vi "save.vi"(0 "ItemNames":string[][](array[string])) -> ()   [LabVIEW 2020]
uses:
  <vilib>/Utility/file.llb/Write Delimited Spreadsheet (string).vi
panel:
  out "Array":string[][](array[string])
  out "error out":errorcluster
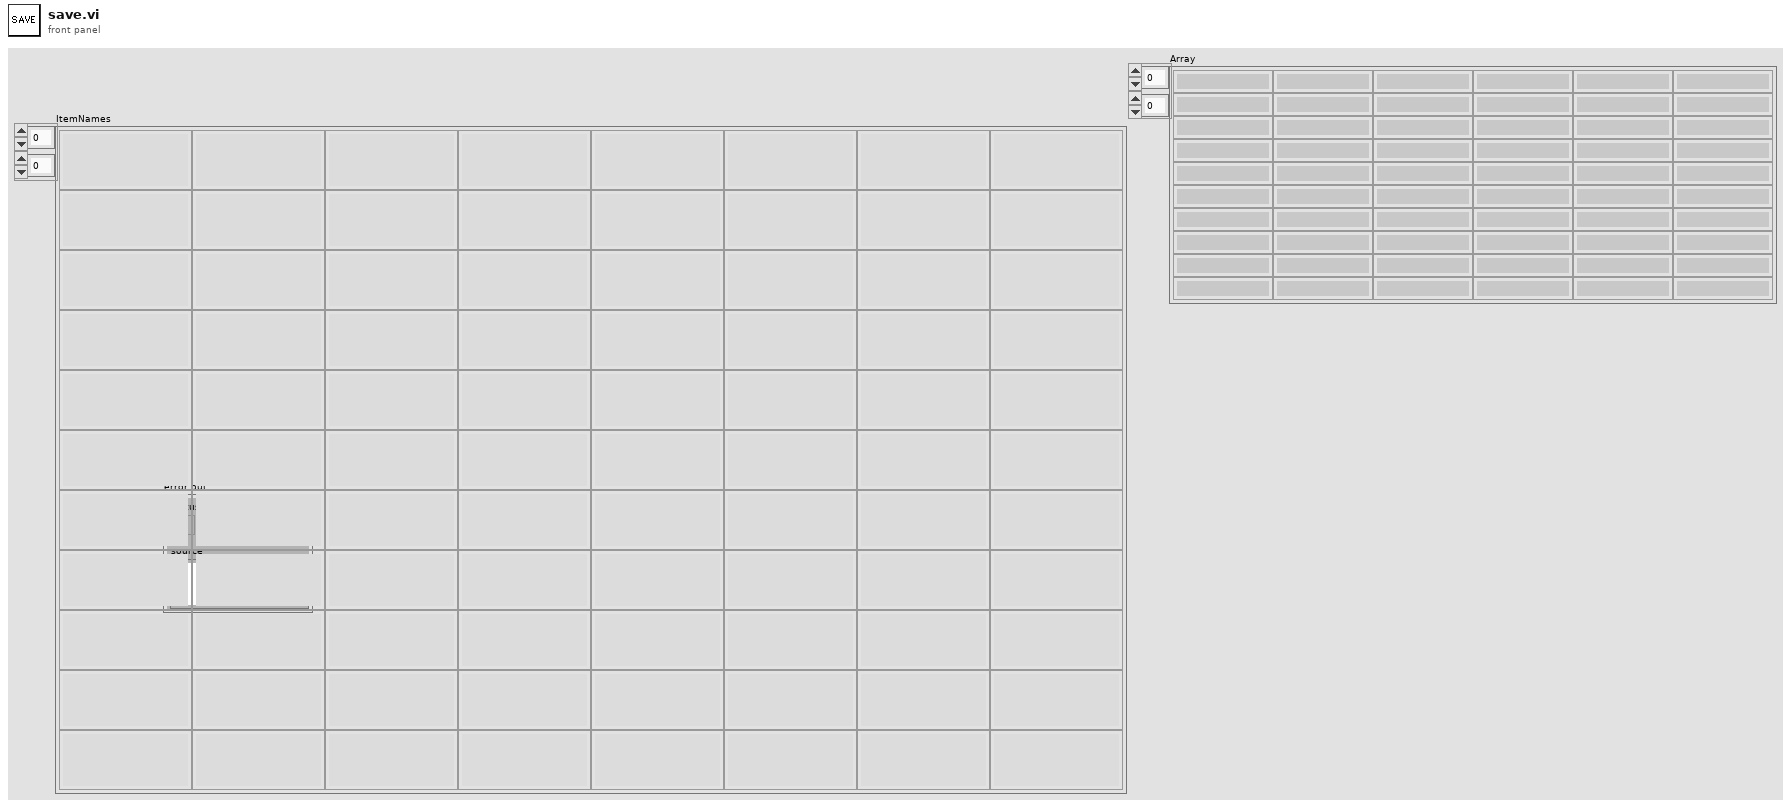
[diagram p1: front panel]
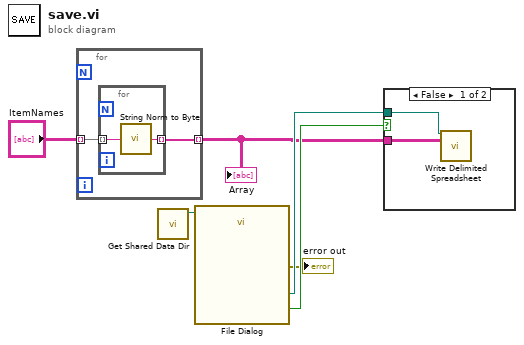
[diagram p0: block diagram]
diagram:
  n1 = for {
    tunnel: "ItemNames" -> [w8] mode=indexing
    tunnel: [w7] -> w1 mode=indexing
    n2 = for {
      tunnel: w8 -> [w10] mode=indexing
      tunnel: [w9] -> w7 mode=indexing
      n3 = call "String Norm to Byte.vi"("String In"=w10) -> ("Byte String Out"=w9:string)
    }
  }
  "Array" <- w1
  n4 = call "Get Shared Data Dir.vi"() -> ("Data Directory Path"=w3:path)  [unwired: 2 in, 1 out]
  n5 = call "File Dialog"("start path"=w3) -> ("selected path"=w5:path, "cancelled"=w6:bool, "error out"=→"error out":errorcluster)  [unwired: 11 in, 1 out]
  n6 = case shown="False" w6 {
    tunnel: w5 -> [w12 _]
    tunnel: w1 -> [w11 _]
    frame False {
      n7 = call-poly <vilib>:"Write Delimited Spreadsheet.vi"("file path (dialog if empty)"=w12, "2D data"=w11) -> ()  [unwired: 12 in, 2 out]
    }
    frame True {
    }
  }
